vi "7-2 hp34401A generatore di funzioni.vi"(0 "N":i32=10, 2 "Limite":dbl format="%.2f", 3 "stop":bool) -> (1 "Tipo di strumento":string, 4 "error out":bool, 5 "Sopra il limite":bool, 6 "vet-dati":dbl[](array[numeric]) format="%.2f", 7 "Max":dbl format="%.2f", 8 "Med":dbl format="%.2f")   [LabVIEW 2012]
doc: "© Copyright M. Ferrari 2003\n Repeated Gpib Measure Exercice & Analisis"
panel:
  out "error code out":i16=-1
  out "Grafico":dbl(graph)
  in  "addr":string="4"
  # "IDENTIFICAZIONE dello STRUMENTO, CONFIGURAZIONE, MISURE RIPETUTE, RAPPRESENTAZIONE dei    \n    VALORI in TEMPO REALE, ANALISI\n    Realizzare un VI che svolga le seguenti funzioni:\n   - richiede l'identificazione dello strumento Hewlett-Packard collegato al bus IEEE 488 e ne visualizza il tipo (es.   34401A) \n   - configura lo strumento per una misura di tensione DC su un range di 1 volt, con una risoluzione di 0.1 mV\n   - effettua un numero N di misure (impostabile da pannello) con un ritardo di 0,5 sec l'una dall'altra, gestendo eventuali \n     errori sull'interfaccia e segnalandone la presenza\n   - visualizza i valori acquisiti su di un grafico in tempo reale e, al termine, li memorizza in un vettore \n   - ricava il valore massimo, il valor medio e verifica (con visualizzazione tramite un indicatore booleano) se almeno uno, tra \n     i valori misurati, supera un valore limite selezionabile da pannello\n   - apportare alla soluzione proposta le modifiche eventualmente necessarie perch sia possibile concludere la misura\n     tramite l'azione, da pannello, su un pulsante di STOP o in caso di errore."
  # "(n¡ misure)"
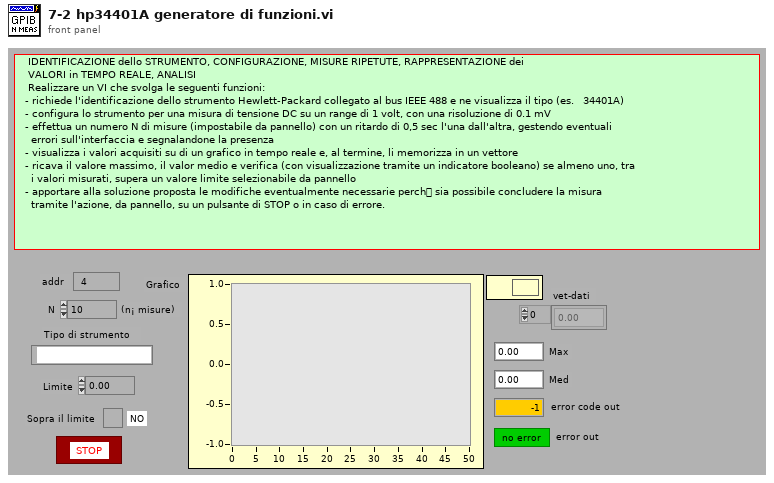
[diagram p1: front panel]
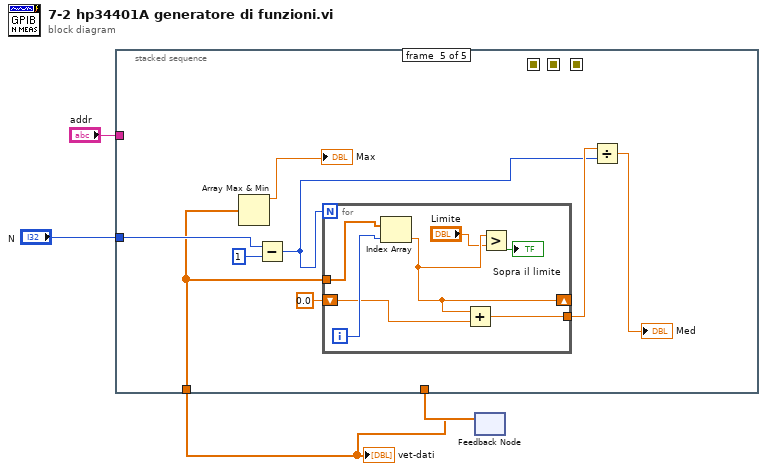
[diagram p0: block diagram]
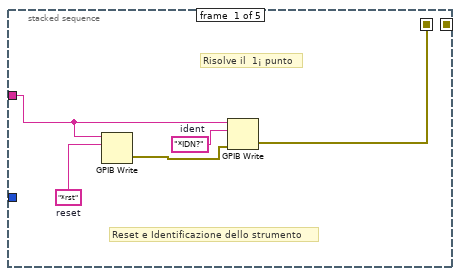
[diagram p2: hidden frame]
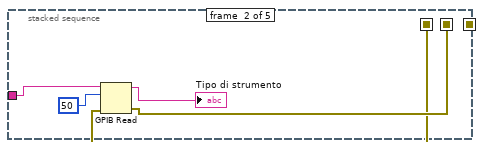
[diagram p3: hidden frame]
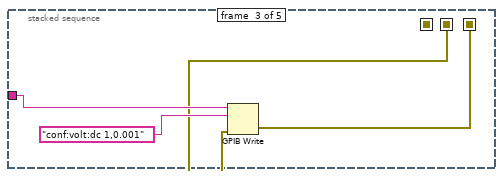
[diagram p4: hidden frame]
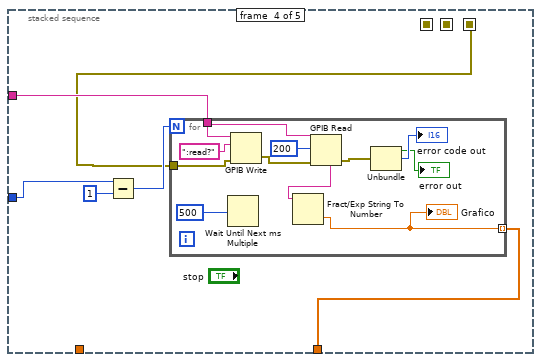
[diagram p5: hidden frame]
diagram:
  n1 = feedback #1() -> (w1:dbl[])  [unwired: 1 in]
  "vet-dati" <- w1
  n2 = stacked-sequence {
    seq-local: [w5 _ _ _ _] -> [_ w10 _ _ _]
    seq-local: [_ w11 _ _ _] -> [_ _ w16 _ _]
    seq-local: [_ _ w15 _ _] -> [_ _ _ w19 _]
    tunnel: "addr" -> [w7 w14 w18 w24 _]
    tunnel: "N" -> [_ _ _ w22 w39]
    tunnel: [_ _ _ w20 _] -> w2
    tunnel: w1 -> [_ _ _ _ w38]
    frame #0 {
      w8 = "*rst"  # reset
      w9 = "*IDN?"  # ident
      # "Reset e Identificazione dello strumento"
      # "Risolve il  1¡ punto"
      n3 = GPIB Write(0:w7, 1:w8) -> (6:w6:errorcluster)  [unwired: 3 in, 1 out]
      n4 = GPIB Write(0:w7, 1:w9, 3:w6) -> (6:w5:errorcluster)  [unwired: 2 in, 1 out]
    }
    frame #1 {
      n5 = GPIB Read(0:w14, 1:50 ("byte count"), 3:w10) -> (5:→"Tipo di strumento":string, 7:w11:errorcluster)  [unwired: 2 in, 1 out]
    }
    frame #2 {
      n6 = GPIB Write(0:w18, 1:"conf:volt:dc 1,0.001" ("data"), 3:w16) -> (6:w15:errorcluster)  [unwired: 2 in, 1 out]
    }
    frame #3 {
      n7 = Subtract(x=w22, y=1) -> (x-y=w21:i32)
      n8 = for {
        N: w21 -> [_]
        tunnel: w24 -> [w35]
        tunnel: [w25] -> w20 mode=indexing
        tunnel: w19 -> [w26]
        n9 = Wait Until Next ms Multiple(millisecond multiple=u32 500 ("millisecond timer value")) -> ()  [unwired: 1 out]
        n10 = GPIB Write(0:w35, 1:":read?" ("address string"), 3:w26) -> (6:w30:errorcluster)  [unwired: 2 in, 1 out]
        n11 = GPIB Read(0:w35, 1:200 ("byte count"), 3:w30) -> (5:w34:string, 7:w29:errorcluster)  [unwired: 2 in, 1 out]
        n12 = Fract/Exp String To Number(string=w34) -> (number=w25:dbl)  [unwired: 3 in, 1 out]
        "Grafico" <- w25
        n13 = Unbundle(w29) -> ("status"=→"error out":bool, "code"=→"error code out":i32)  [unwired: 1 out]
      }
    }
    frame #4 {
      n14 = Array Max & Min(array=w38) -> (max value=→"Max":dbl)  [unwired: 3 out]
      n15 = Subtract(x=w39, y=1) -> (x-y=w41:i32)
      n16 = for {
        N: w41 -> [_]
        shift-right: [w45] -> _
        shift-left: 0.0 -> [w48]
        tunnel: w38 -> [w50]
        tunnel: [w47] -> w42
        i -> [w49]
        n17 = Index Array(array=w50, index=w49) -> (element=w45:dbl)
        n18 = Add(x=w45, y=w48) -> (x+y=w47:dbl)
        n19 = Greater?(x=w45, y="Limite") -> (0:→"Sopra il limite":bool)
      }
      n20 = Divide(x=w42, y=w41) -> (x/y=→"Med":dbl)
    }
  }
  n21 = feedback-in #1(w2) -> ()
